vi "Panel.vi"(11 "AppListPanel in":refnum<class "AppListPanel.lvclass">) -> ()   [LabVIEW 2020, in "PicoG-App.lvlib" / "AppListPanel.lvclass"]
uses:
  AppListPanel.lvclass
  C:/Program Files (x86)/National Instruments/LabVIEW 2020/vi.lib/IlluminatedG/IG OOPanel/OOPanel/Panel/Panel.lvclass
  <vilib>/IlluminatedG/IG OOPanel/OOPanel/Panel/Basic UI State.ctl
  AppListPanel.lvclass/AppListPanel.ctl
  ViaApp/ViaApp.lvclass
  <vilib>/IlluminatedG/IG OOPanel/OOPanel/Panel/Panel.lvclass
  <vilib>/IlluminatedG/IG OOPanel/OOPanel/OOPanel.lvlib
  <vilib>/IlluminatedG/IG OOPanel/OOPanel/ArrayManager/ArrayManager.lvclass
  App/App.lvclass
  C:/dev/Vireo/PicoG/PicoG-App/NavPanel/NavPanel.lvclass
  C:/dev/Vireo/PicoG/PicoG-App/AppListPanel/AppListPanel.lvclass
  Sort Order.ctl
panel:
  in  "Sort Order":T1
  in  "Add":bool
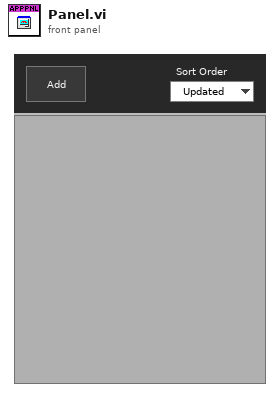
[diagram p1: front panel]
types:
  T1 = typedef "PicoG-App.lvlib/AppListPanel.lvclass/Sort Order.ctl" = enum16{"Updated", "Name"}
  T2 = typedef "OOPanel.lvlib/Panel.lvclass/Basic UI State.ctl" = enum16{"Init", "Run", "Close"}
  T3 = enum32{"Invalid", "Standard", "Closed", "Hidden", "Minimized", "Maximized"}
  T4 = typedef "PicoG-App.lvlib/AppListPanel.lvclass/Panel Events.ctl" = cluster{"Update App":refnum<user-event>}
  T5 = typedef "OOPanel.lvlib/Panel.lvclass/Panel Events.ctl" = cluster{"Visbility":refnum<user-event>, "Close":refnum<user-event>}
  T6 = typedef "PicoG-App.lvlib/AppListPanel.lvclass/Ref Data.ctl" = cluster{"App Map":map{path, refnum<class "ViaApp.lvclass">}}
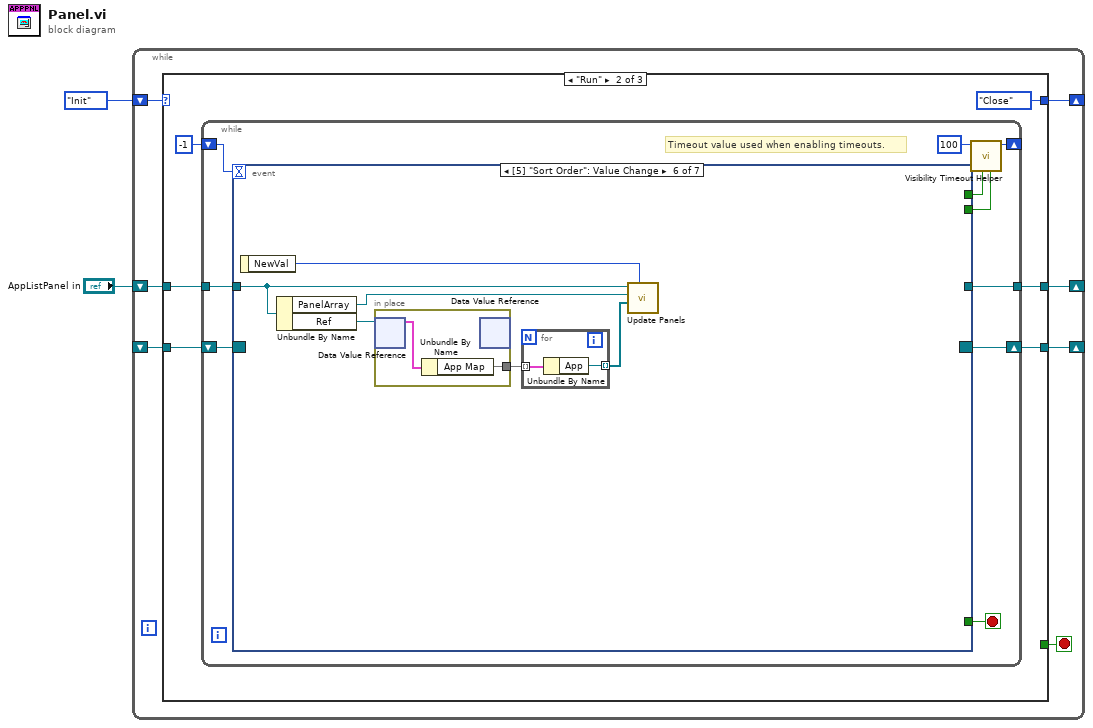
[diagram p0: block diagram]
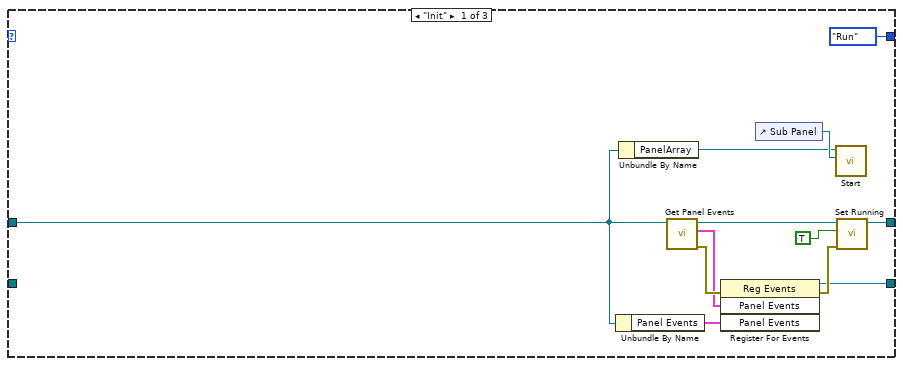
[diagram p2: hidden frame]
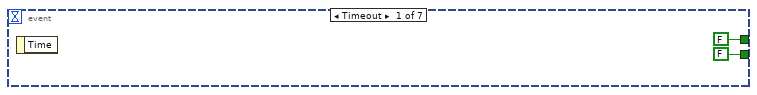
[diagram p3: hidden frame]
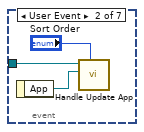
[diagram p4: hidden frame]
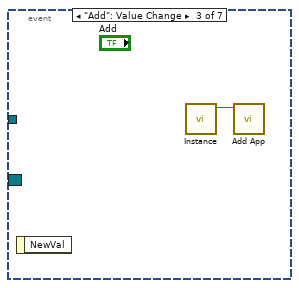
[diagram p5: hidden frame]
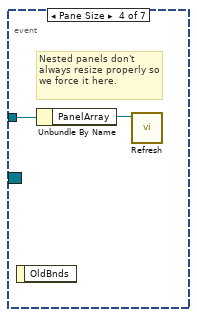
[diagram p6: hidden frame]
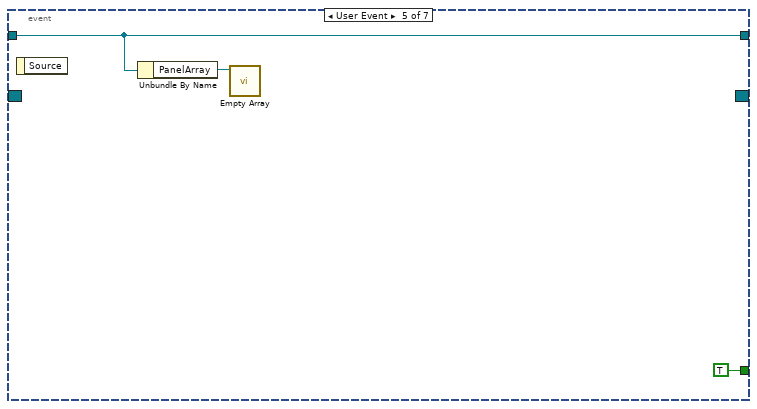
[diagram p7: hidden frame]
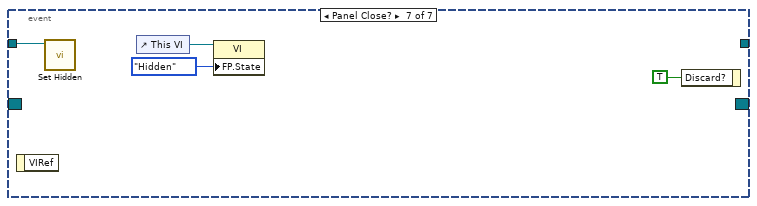
[diagram p8: hidden frame]
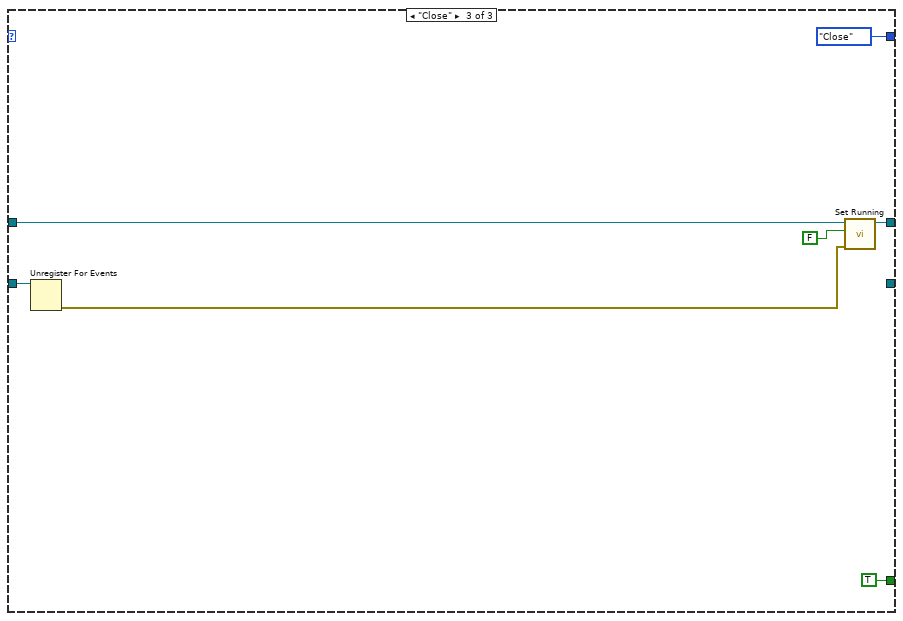
[diagram p9: hidden frame]
diagram:
  n1 = while {
    shift-right: [w8] -> _
    shift-left: _ -> [w9]
    shift-right: [w6] -> _
    shift-left: Basic_UI_State."Init" ("Basic UI State") -> [w7]
    shift-right: [w4] -> _
    shift-left: "AppListPanel in" -> [w3]
    stop <- w5 stop-if-true
    n2 = case shown="\"Run\"" w7 {
      tunnel: w9 -> [_ w27 w65]
      tunnel: [w15 w25 _] -> w8
      tunnel: [Basic_UI_State."Run" ("Basic UI State") Basic_UI_State."Close" ("Basic UI State") Basic_UI_State."Close" ("Basic UI State")] -> w6
      tunnel: [_ _ TRUE] -> w5
      tunnel: [w14 w22 w63] -> w4
      tunnel: w3 -> [w10 w23 w64]
      frame "Init" {
        n3 = Unbundle By Name(w10) -> ("Panel Events"=w11:T4)
        n4 = Unbundle By Name(w10) -> ("PanelArray"=w12:refnum<class "ArrayManager.lvclass">)
        n5 = call <vilib>:"Get Panel Events.vi"("Panel in"=w10) -> ("error out"=w21:errorcluster, "Panel Events"=w17:T5, "Panel out"=w18:refnum<class "AppListPanel.lvclass">)  [unwired: 8 in]
        n6 = register-events(error in=w21, w17, w11) -> (reference out=w15:refnum<event-registration>, error out=w19:errorcluster)  [unwired: 1 in]
        n7 = control-ref of="Sub Panel"() -> (w13:refnum<vi>)
        n8 = call <vilib>:"Start.vi"("Container"=w13, "ArrayManager in"=w12) -> ()  [unwired: 8 in, 2 out]
        n9 = call <vilib>:"Set Running.vi"("error in (no error)"=w19, "Running"=TRUE, "Panel in"=w18) -> ("Panel out"=w14:refnum<class "AppListPanel.lvclass">)  [unwired: 7 in, 1 out]
      }
      frame "Run" {
        n10 = while {
          shift-right: [w33] -> w25
          shift-left: w27 -> [w34]
          shift-right: [w36] -> _
          shift-left: -1 ("Timeout") -> [w35]
          tunnel: w23 -> [w29]
          tunnel: [w28] -> w22
          stop <- w30 stop-if-true
          # "Timeout value used when enabling timeouts."
          n11 = event shown="[5] \"Sort Order\": Value Change" {
            selector: w34 -> [_ _ _ _ _ _ _]
            dyn-events: [_ _ _ _ _ _ _] -> w33
            timeout: w35 -> [_ _ _ _ _ _ _]
            tunnel: [FALSE _ _ _ _ _ _] -> w32
            tunnel: [FALSE _ _ _ _ _ _] -> w31
            tunnel: [_ _ _ _ TRUE _ _] -> w30
            tunnel: w29 -> [_ w42 _ w45 w47 w52 w59]
            tunnel: [_ _ _ _ w47 _ _] -> w28
            event Timeout {
              n12 = event-data() -> ()  [unwired: 1 in, 1 out]
            }
            event User Event {
              n13 = event-data() -> ("App"=w41:refnum<class "ViaApp.lvclass">)  [unwired: 1 in]
              n14 = call "Handle Update App.vi"("Sort Order"="Sort Order", "ViaApp"=w41, "AppListPanel in"=w42) -> ()  [unwired: 7 in, 2 out]
            }
            event "Add": Value Change {
              n15 = event-data() -> ()  [unwired: 1 in, 1 out]
              n16 = call "Instance.vi"() -> ("App out"=w43:refnum<class "App.lvclass">)  [unwired: 10 in, 1 out]
              n17 = call "Add App.vi"("App in"=w43) -> ()  [unwired: 9 in, 2 out]
            }
            event Pane Size {
              # "Nested panels don't always resize properly so we force it here."
              n18 = event-data() -> ()  [unwired: 1 in, 1 out]
              n19 = Unbundle By Name(w45) -> ("PanelArray"=w44:refnum<class "ArrayManager.lvclass">)
              n20 = call <vilib>:"Refresh.vi"("ArrayManager in"=w44) -> ()  [unwired: 9 in, 2 out]
            }
            event User Event {
              n21 = event-data() -> ()  [unwired: 1 in, 1 out]
              n22 = Unbundle By Name(w47) -> ("PanelArray"=w46:refnum<class "ArrayManager.lvclass">)
              n23 = call <vilib>:"Empty Array.vi"("ArrayManager in"=w46) -> ()  [unwired: 9 in, 2 out]
            }
            event Value Change {
              n24 = event-data() -> ("NewVal"=w54:T1)  [unwired: 1 in]
              n25 = Unbundle By Name(w52) -> ("PanelArray"=w49:refnum<class "ArrayManager.lvclass">, "Ref"=w53:refnum<data-value>)
              n26 = in-place {
                in-place-border: [w57] -> w51
                n27 = in-place-dvr #1(w53) -> (w58:T6)  [unwired: 1 out]
                n28 = Unbundle By Name(w58) -> ("App Map"=w57:map{path, refnum<class "ViaApp.lvclass">})
                n29 = in-place-dvr #1() -> ()  [unwired: 1 in, 2 out]
              }
              n30 = for {
                tunnel: w51 -> [w56] mode=indexing
                tunnel: [w55] -> w50 mode=indexing
                n31 = Unbundle By Name(w56) -> ("App"=w55:refnum<class "ViaApp.lvclass">)
              }
              n32 = call "Update Panels.vi"("Sort Order"=w54, "Apps"=w50, "PanelArray"=w49, "AppListPanel"=w52) -> ()  [unwired: 8 in]
            }
            event Panel Close? {
              n33 = event-data() -> ()  [unwired: 1 in, 1 out]
              n34 = call <vilib>:"Set Hidden.vi"("Panel in"=w59) -> ()  [unwired: 9 in, 2 out]
              n35 = control-ref of="This VI"() -> (w61:refnum<vi>)
              n36 = property class="VI"(reference=w61, "FP.State"=T3."Hidden" ("Front Panel Window:State")) -> ()  [unwired: 1 in, 2 out]
              n37 = event-data("Discard?"=TRUE) -> ()  [unwired: 1 in, 1 out]
            }
          }
          n38 = call <vilib>:"Visibility Timeout Helper.vi"("Update?"=w31, "Use Timeout?"=w32, "Visible Timeout mS"=100) -> ("Timeout"=w36:i32)  [unwired: 8 in]
        }
      }
      frame "Close" {
        n39 = Unregister For Events(event registration refnum=w65) -> (error out=w67:errorcluster)  [unwired: 1 in]
        n40 = call <vilib>:"Set Running.vi"("error in (no error)"=w67, "Running"=FALSE, "Panel in"=w64) -> ("Panel out"=w63:refnum<class "AppListPanel.lvclass">)  [unwired: 7 in, 1 out]
      }
    }
  }
